vi "Select Platform UI.vi"(8 "error in (no error)":errorcluster, 11 "Plugins":refnum<class "PlatformPluginManager.lvclass">) -> (0 "error out":errorcluster, 2 "Cancelled":bool, 3 "Platform":string)   [LabVIEW 2020, in "PicoG-App.lvlib" / "App.lvclass"]
uses:
  App.lvclass
  Builds/picoG/ppl/PicoG-Core.lvlibp/PicoG-Processor/PicoG-Core/PlatformPluginManager/PlatformPluginManager.lvclass
panel:
  in  "Cancel":bool
  in  "OK":bool
  in  "Select Platform":string(combo)
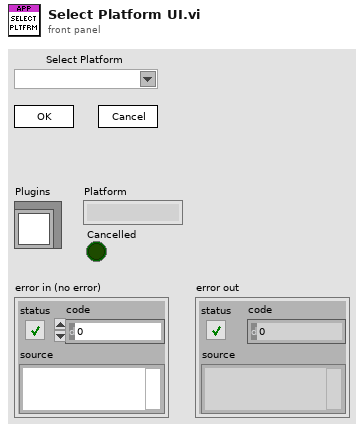
[diagram p1: front panel]
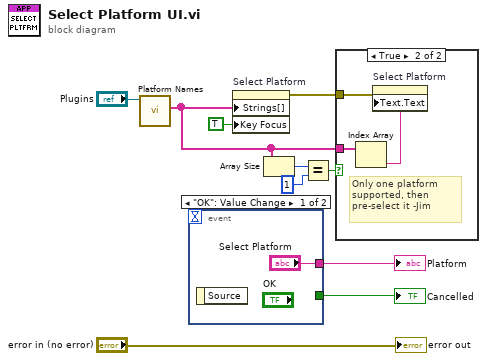
[diagram p0: block diagram]
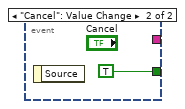
[diagram p3: hidden frame]
diagram:
  n1 = call "Platform Names.vi"("TargetPluginManager in"="Plugins") -> ("Platforms"=w3:string[])  [unwired: 8 in, 2 out]
  n2 = event shown="[0] \"OK\": Value Change" {
    selector: _ -> [_ _]
    dyn-events: _ -> [_ _]
    timeout: _ -> [_ _]
    tunnel: ["Select Platform" _] -> w9
    tunnel: [_ TRUE] -> w8
    event "OK": Value Change {
      n3 = event-data() -> ()  [unwired: 1 in, 1 out]
    }
    event "Cancel": Value Change {
      n4 = event-data() -> ()  [unwired: 1 in, 1 out]
    }
  }
  "Platform" <- w9
  "Cancelled" <- w8
  n5 = property on="Select Platform" class="CmbBox"("Strings[]"=w3, "Key Focus"=TRUE) -> (error out=w4:errorcluster)  [unwired: 2 in, 1 out]
  n6 = Array Size(array=w3) -> (size(s)=w7:i32)
  n7 = Equal?(x=w7, y=1) -> (x = y?=w5:bool)
  n8 = case shown="True" w5 {
    tunnel: w4 -> [_ w15]
    tunnel: w3 -> [_ w14]
    frame False {
    }
    frame True {
      # "Only one platform supported, then pre-select it -Jim"
      n9 = Index Array(array=w14) -> (element=w13:string)  [unwired: 1 in]
      n10 = property on="Select Platform" class="CmbBox"(error in=w15, "Text.Text"=w13) -> ()  [unwired: 1 in, 2 out]
    }
  }
  "error out" <- "error in (no error)"
